vi "A1343 4 nibble calc CRC (1).vi"(0 "Data":u8[](array[numeric])=[7, 15, 15, 0] format="%x") -> (4 "CRC":u8 format="%x")   [LabVIEW 2013]
doc: "This VI calculates the checksum required for outgoing and incoming SENT data."
panel:
  out "size(s) 2":i32
  out "size(s)":i32
  out "Numeric":i32
  # "CRC-4"
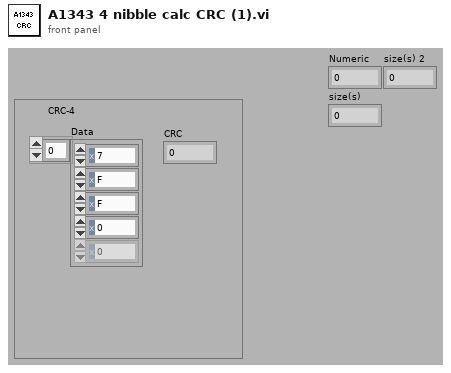
[diagram p1: front panel]
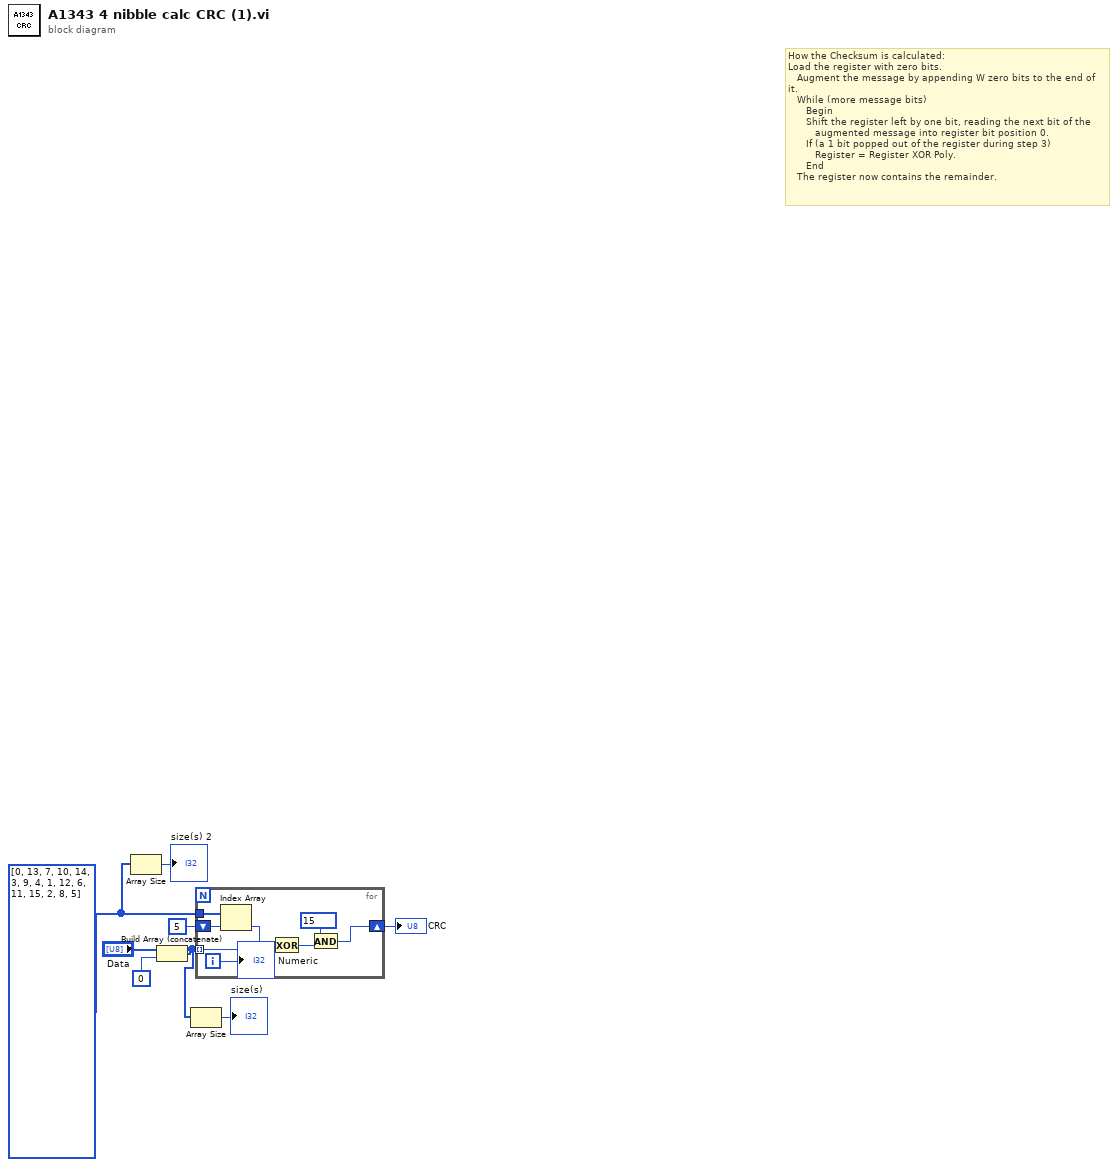
[diagram p0: block diagram]
diagram:
  w2 = u8[] [0, 13, 7, 10, 14, 3, 9, 4, 1, 12, 6, 11, 15, 2, 8, 5] ("Data 4")
  # "How the Checksum is calculated:\nLoad the register with zero bits.\n   Augment the message by appending W zero bits to the end of it.\n   While (more message bits)\n      Begin\n      Shift the register left by one bit, reading the next bit of the\n         augmented message into register bit position 0.\n      If (a 1 bit popped out of the register during step 3)\n         Register = Register XOR Poly.\n      End\n   The register now contains the remainder."
  n1 = Array Size(array=w2) -> (size(s)=→"size(s) 2":i32)
  n2 = Build Array (concatenate)("Data", u8 0) -> (w4:u8[])
  n3 = Array Size(array=w4) -> (size(s)=→"size(s)":i32)
  n4 = for {
    tunnel: w4 -> [w15] mode=indexing
    shift-right: [w11] -> w6
    shift-left: u8 5 ("x") -> [w10]
    tunnel: w2 -> [w16]
    i -> [w9]
    n5 = Index Array(array=w16, index=w10) -> (element=w14:u8)
    n6 = Exclusive Or(1:w15, 2:w14) -> (0:w12:u8)
    n7 = And(x=u8 15, y=w12) -> (x .and. y?=w11:u8)
    "Numeric" <- w9
  }
  "CRC" <- w6
